vi "DropTable.vi"(10 "Table Name":string, 11 "Path":path) -> (1 "OK？":bool, 2 "Table Name":string, 3 "Path":path)   [LabVIEW 2017, in "SQLite.lvlib"]
uses:
  SQLite.lvlib
  Core/Tables/SQLite_Drop Table.vi
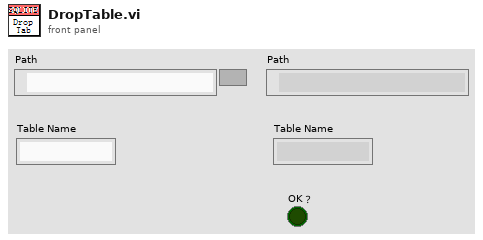
[diagram p1: front panel]
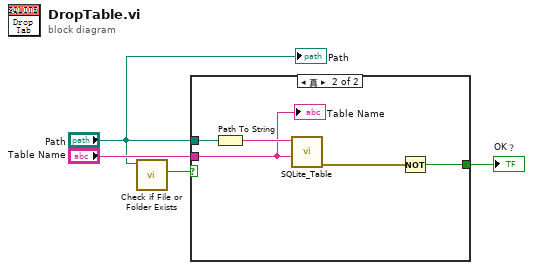
[diagram p0: block diagram]
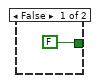
[diagram p2: hidden frame]
diagram:
  n1 = call <vilib>:"Check if File or Folder Exists.vi"("path"="Path") -> ("file or folder exists?"=w1:bool)  [unwired: 8 in, 2 out]
  n2 = case shown="真" w1 {
    tunnel: [FALSE w8] -> w4
    tunnel: "Table Name" -> [_ w7]
    tunnel: "Path" -> [_ w6]
    frame False {
    }
    frame True {
      n3 = Path To String(path=w6) -> (string=w10:string)
      n4 = call-poly "SQLite_Table.vi"("DB Path"=w10, "Table Name"=w7) -> ("error out"=w9:errorcluster)  [unwired: 6 in, 2 out]
      n5 = Not(x=w9) -> (.not. x?=w8:bool)
      "Table Name" <- w7
    }
  }
  "OK？" <- w4
  "Path" <- "Path"
